vi "DO Control.vi"(9 "DI List_280":string[](array[string]), 10 "s":bool, 11 "DO":T1) -> (0 "Feedback":i32[](array[numeric]), 1 "Parameter (Out)":u8 caption="Poll Type", 2 "Control Channel 2":i32[](array[numeric]), 3 "Poll Time (Out)":u32 caption="Poll Time (ms)" max=600000 step=100, 4 "Value":enum32{"Output", "Input"}(ring), 5 "Cancel":bool)   [LabVIEW 2015]
uses:
  Control Button/Exit.ctl
  Control Button/next.ctl
  Control PB/output control.ctl
  Data Acquisition/PCI-USB-DAQ/Digital out put.ctl
  Galobal variable_TI.vi
panel:
  out "Row":i32
  in  "s 2":bool
  out "Pokayoka Result":cluster{"Sensor Name":string, "Boolean":bool}[](array[cluster]) caption="Pokayoka Status"
  in  "Tab Control":enum32{"Output", "Input"}(tab)
  in  "Control Channel":i32[](listbox)=[7]
  in  "op Add":T2
  in  "Feed Back Channel":i32[](listbox)=[0]
  in  "ok":T3
  in  "stop":T4
  # "Control Channel"
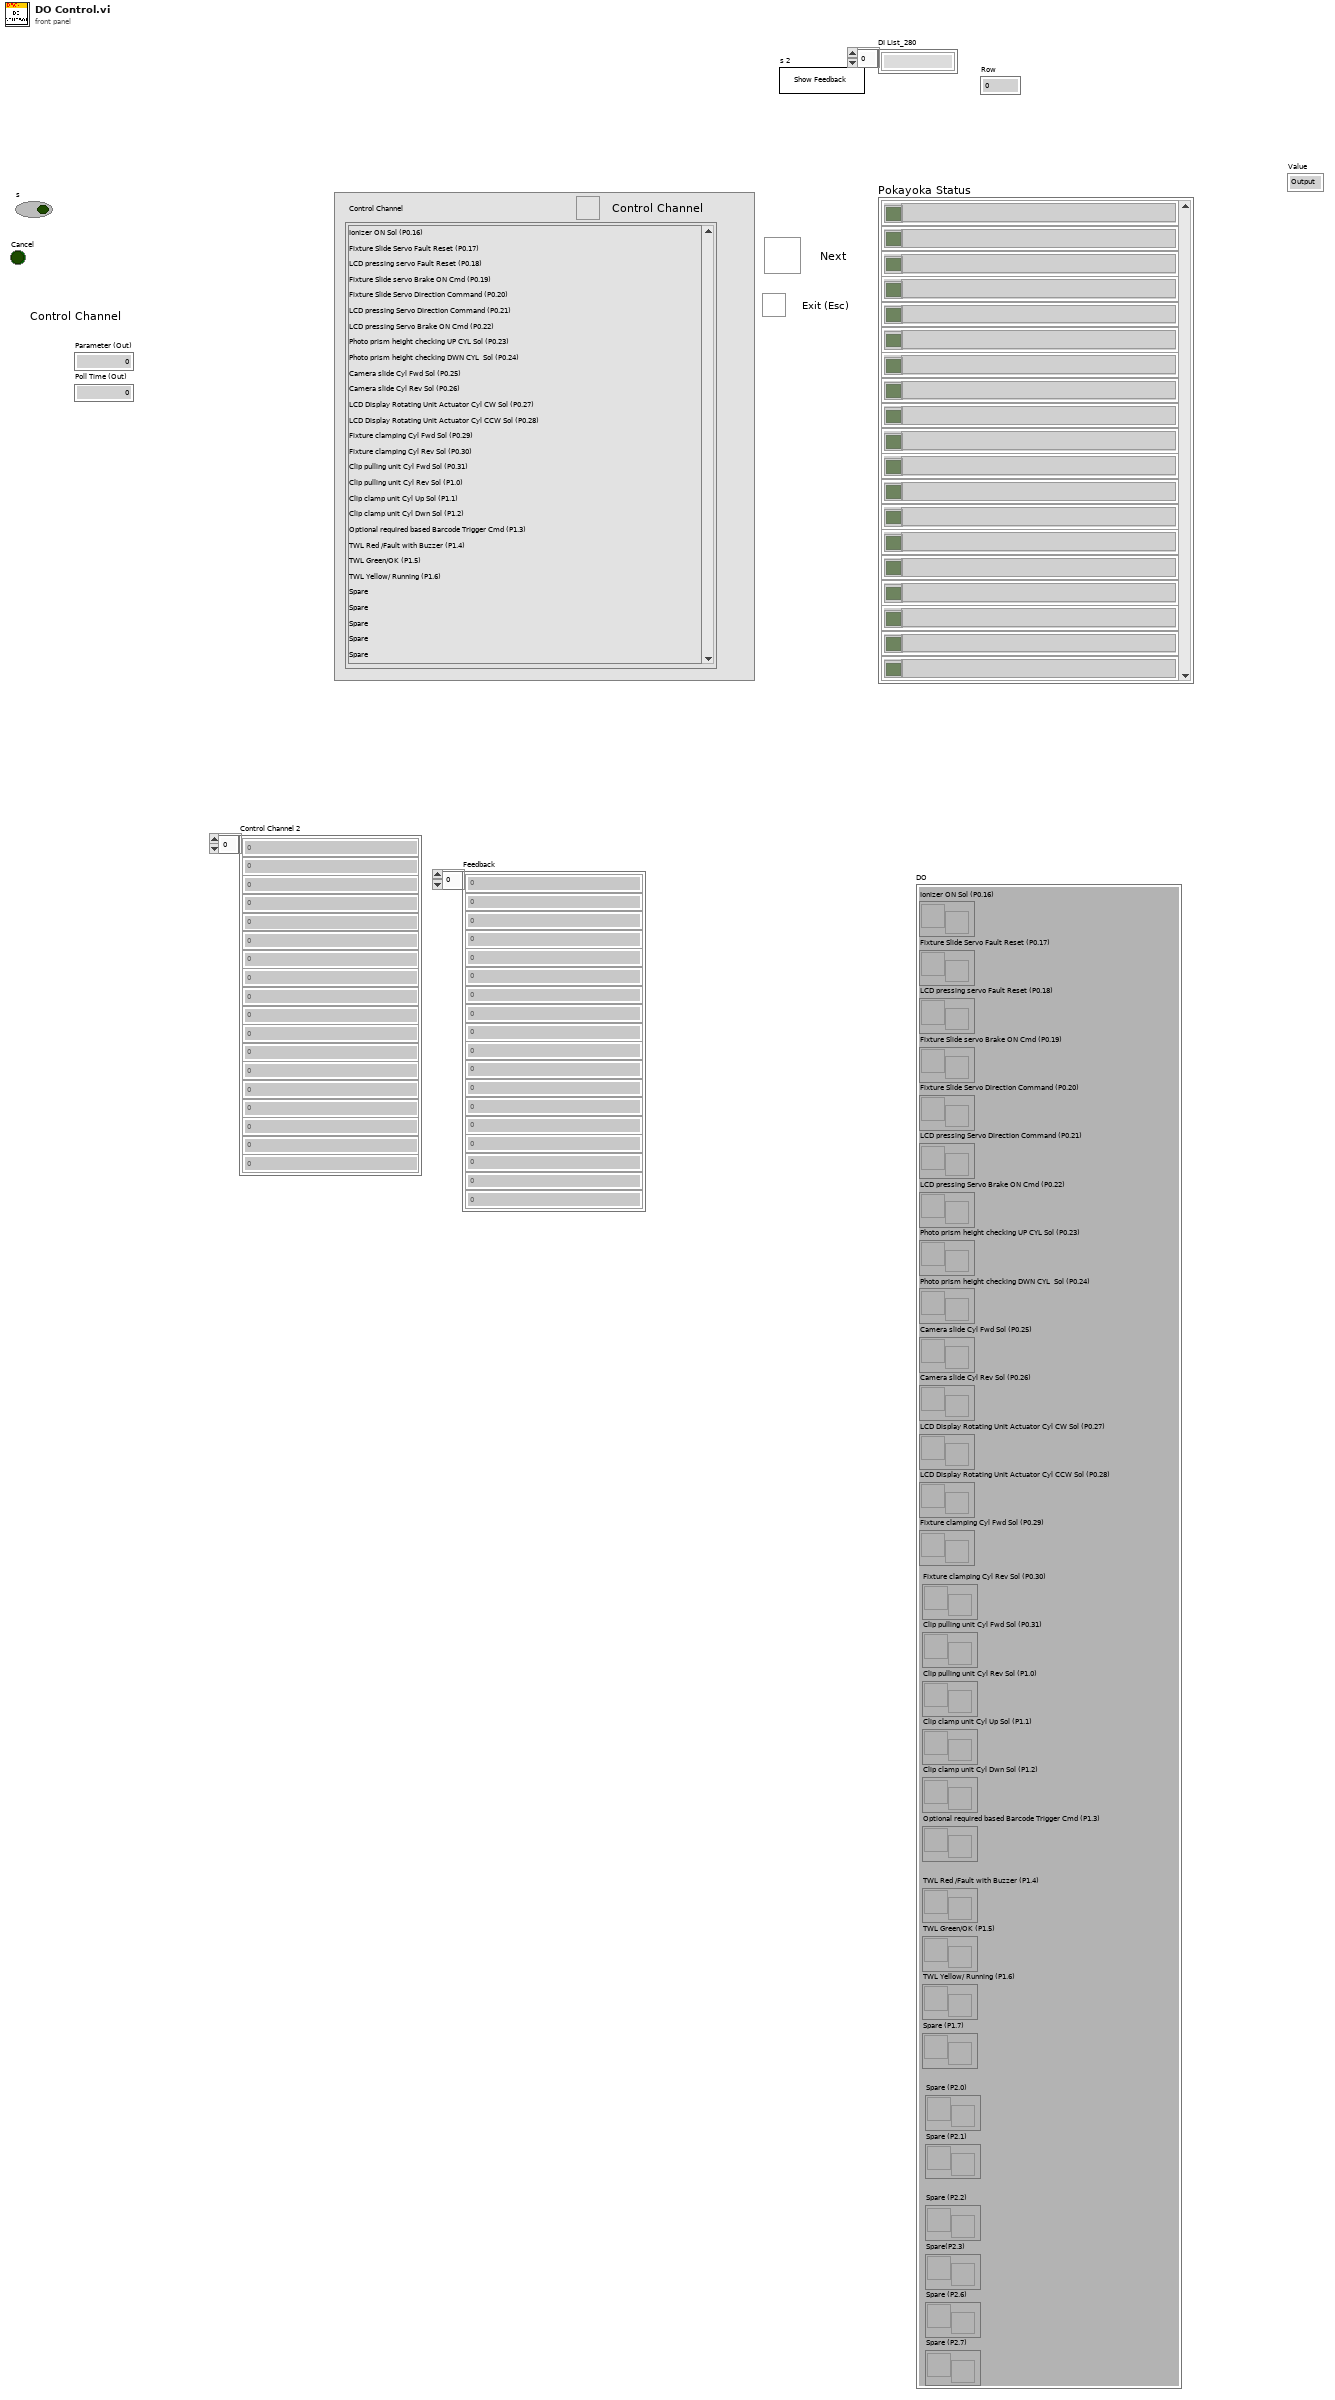
[diagram p1: front panel]
types:
  T1 = typedef "Digital out put.ctl" = cluster{"Ionizer ON Sol (P0.16)":refnum<notifier>, "Fixture Slide Servo Fault Reset (P0.17)":refnum<notifier>, "LCD pressing servo Fault Reset (P0.18)":refnum<notifier>, "Fixture Slide servo Brake ON Cmd (P0.19)":refnum<notifier>, "Fixture Slide Servo Direction Command (P0.20)":refnum<notifier>, "LCD pressing Servo Direction Command (P0.21)":refnum<notifier>, "LCD pressing Servo Brake ON Cmd (P0.22)":refnum<notifier>, "Photo prism height checking UP CYL Sol (P0.23)":refnum<notifier>, "Photo prism height checking DWN CYL  Sol (P0.24)":refnum<notifier>, "Camera slide Cyl Fwd Sol (P0.25)":refnum<notifier>, "Camera slide Cyl Rev Sol (P0.26)":refnum<notifier>, "LCD Display Rotating Unit Actuator Cyl CW Sol (P0.27)":refnum<notifier>, "LCD Display Rotating Unit Actuator Cyl CCW Sol (P0.28)":refnum<notifier>, "Fixture clamping Cyl Fwd Sol (P0.29)":refnum<notifier>, "Fixture clamping Cyl Rev Sol (P0.30)":refnum<notifier>, "Clip pulling unit Cyl Fwd Sol (P0.31)":refnum<notifier>, "Clip pulling unit Cyl Rev Sol (P1.0)":refnum<notifier>, "Clip clamp unit Cyl Up Sol (P1.1)":refnum<notifier>, "Clip clamp unit Cyl Dwn Sol (P1.2)":refnum<notifier>, "Optional required based Barcode Trigger Cmd (P1.3)":refnum<notifier>, "TWL Red /Fault with Buzzer (P1.4)":refnum<notifier>, "TWL Green/OK (P1.5)":refnum<notifier>, "TWL Yellow/ Running (P1.6)":refnum<notifier>, "Spare (P1.7)":refnum<notifier>, "Spare (P2.0)":refnum<notifier>, "Spare (P2.1)":refnum<notifier>, "Spare (P2.2)":refnum<notifier>, "Spare(P2.3)":refnum<notifier>, "Spare (P2.6)":refnum<notifier>, "Spare (P2.7) ":refnum<notifier>}
  T2 = typedef "output control.ctl" = bool
  T3 = typedef "next.ctl" = bool
  T4 = typedef "Exit.ctl" = bool
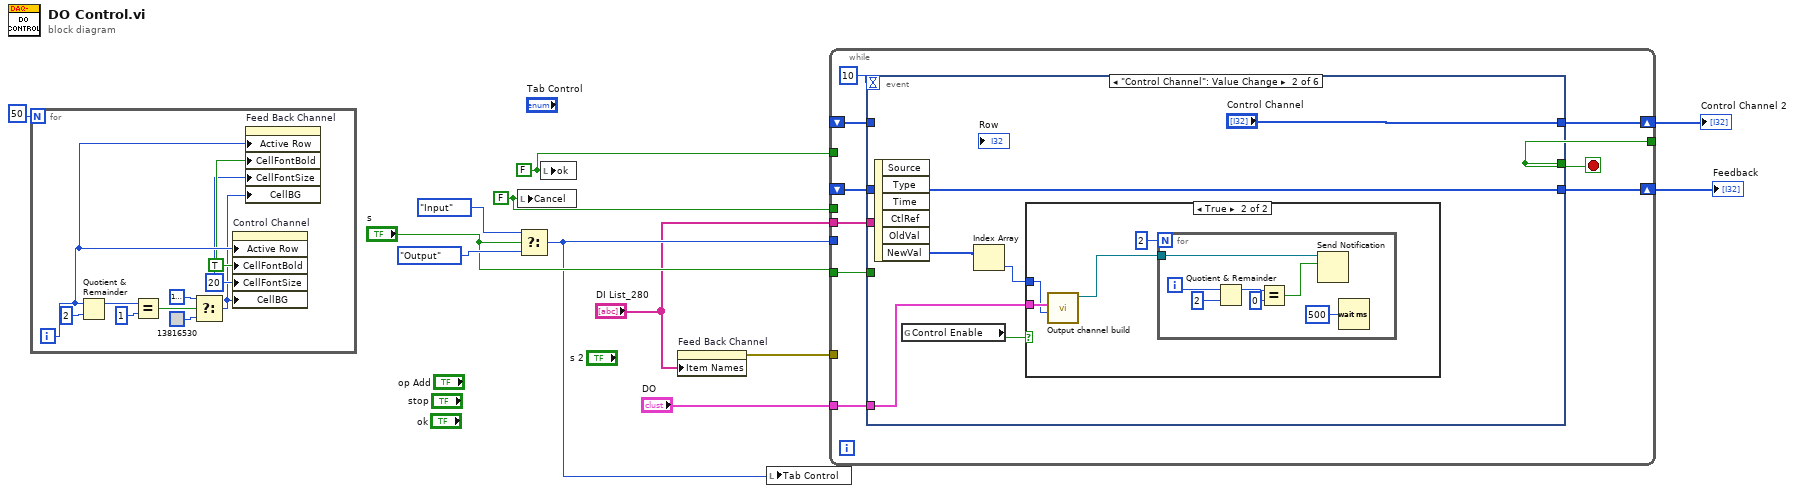
[diagram p0: block diagram]
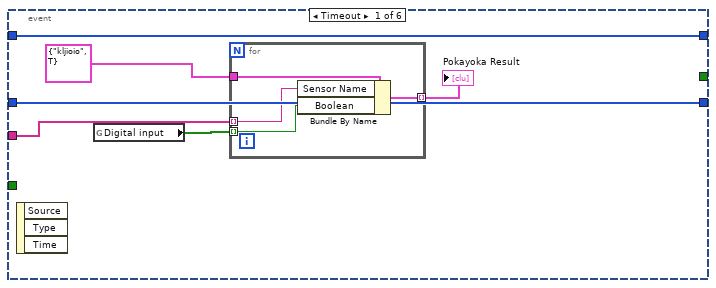
[diagram p2: hidden frame]
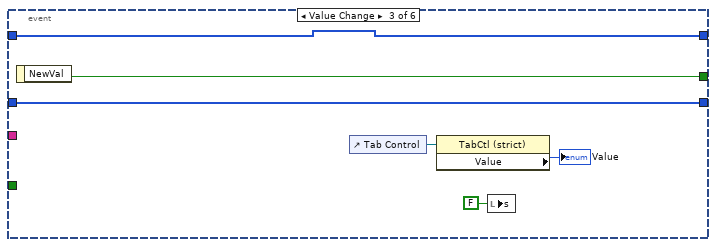
[diagram p4: hidden frame]
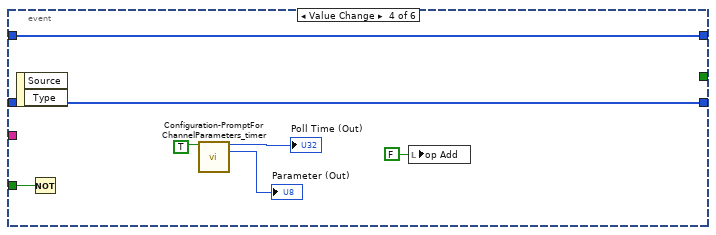
[diagram p5: hidden frame]
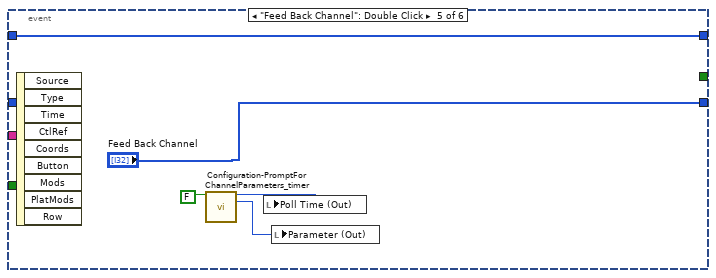
[diagram p6: hidden frame]
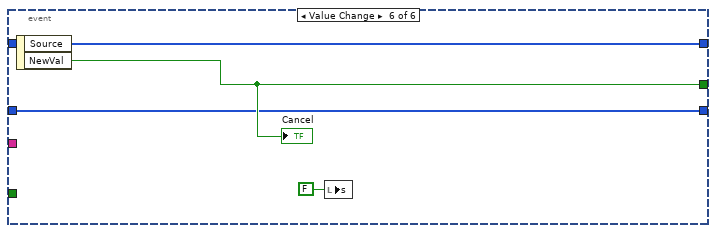
[diagram p7: hidden frame]
diagram:
  w5 = FALSE ("Cancel")
  w6 = FALSE ("ok")
  n1 = for {
    N: 50 -> [_]
    i -> [w16]
    w14 = u32 20 ("Active Row:Cell Font:Size")
    w15 = TRUE ("Active Row:Cell Font:Bold")
    n2 = Quotient & Remainder(x=w16, y=2) -> (x-y*floor(x/y)=w21:i32)  [unwired: 1 out]
    n3 = Equal?(x=w21, y=1) -> (x = y?=w19:bool)
    n4 = Select(t=u32 16777225 ("Color Box"), s=w19, f=u32 13816530 ("Color Box")) -> (s? t:f=w13:u32)
    n5 = property on="Control Channel" class="LstBox (strict)"("Active Row"=w16, "CellFontBold"=w15, "CellFontSize"=w14, "CellBG"=w13) -> ()  [unwired: 2 in, 2 out]
    n6 = property on="Feed Back Channel" class="LstBox (strict)"("Active Row"=w16, "CellFontBold"=w15, "CellFontSize"=w14, "CellBG"=w13) -> ()  [unwired: 2 in, 2 out]
  }
  n7 = local write "Cancel"(w5) -> ()
  n8 = Select(t=enum32{"Output", "Input"}."Input" ("Tab Control"), s="s", f=enum32{"Output", "Input"}."Output" ("Tab Control")) -> (s? t:f=w8:enum32{"Output", "Input"})
  n9 = local write "ok"(w6) -> ()
  n10 = property on="Feed Back Channel" class="LstBox (strict)"("Item Names"="DI List_280") -> (error out=w3:errorcluster)  [unwired: 2 in, 1 out]
  n11 = local write "Tab Control"(w8) -> ()
  n12 = while {
    tunnel: w8 -> [_]
    tunnel: "s" -> [w30]
    tunnel: w6 -> [_]
    tunnel: [w28] -> _
    tunnel: w5 -> [_]
    shift-right: [w31] -> w12
    shift-left: _ -> [w27]
    shift-right: [w29] -> w7
    shift-left: _ -> [w26]
    tunnel: "DI List_280" -> [w25]
    tunnel: w3 -> [_]
    tunnel: "DO" -> [w23]
    stop <- w28 stop-if-true
    n13 = event shown="[1] \"Control Channel\": Value Change" {
      selector: _ -> [_ _ _ _ _ _]
      dyn-events: _ -> [_ _ _ _ _ _]
      timeout: 10 -> [_ _ _ _ _ _]
      tunnel: [w37 "Control Channel" w60 w69 w73 w78] -> w31
      tunnel: [_ _ w64 _ _ w79] -> w28
      tunnel: w30 -> [_ _ _ w70 _ _]
      tunnel: [w36 w46 w59 w68 "Feed Back Channel" w77] -> w29
      tunnel: w27 -> [w37 _ w60 w69 w73 w78]
      tunnel: w26 -> [w36 w46 w59 w68 _ w77]
      tunnel: w25 -> [w33 _ _ _ _ _]
      tunnel: w23 -> [_ w43 _ _ _ _]
      event Timeout {
        n14 = event-data() -> ()  [unwired: 1 in, 3 out]
        n15 = global read "Galobal variable_TI.vi" "Digital input"() -> (w35:bool[])
        n16 = for {
          tunnel: w33 -> [w40] mode=indexing
          tunnel: cluster{"Sensor Name":string, "Boolean":bool} {"Sensor Name"="kljioio", "Boolean"=TRUE} ("Cluster") -> [w41]
          tunnel: [w39] -> w32 mode=indexing
          tunnel: w35 -> [w38] mode=indexing
          n17 = Bundle By Name(cluster=w41, "Sensor Name"=w40, "Boolean"=w38) -> (w39:cluster{"Sensor Name":string, "Boolean":bool})
        }
        "Pokayoka Result" <- w32
      }
      event "Control Channel": Value Change {
        n18 = event-data() -> ("NewVal"=w45:i32[])  [unwired: 1 in, 5 out]
        n19 = global read "Galobal variable_TI.vi" "Control Enable"() -> (w42:bool)
        n20 = Index Array(array=w45) -> (element=w44:i32)  [unwired: 1 in]
        n21 = case shown="True" w42 {
          tunnel: w44 -> [_ w50]
          tunnel: w43 -> [_ w51]
          frame False {
          }
          frame True {
            n22 = call "Output channel build.vi"("Channel No"=w50, "DO"=w51) -> ("Output channel"=w48:refnum<notifier>)  [unwired: 9 in]
            n23 = for {
              N: 2 -> [_]
              tunnel: w48 -> [w52]
              i -> [w58]
              n24 = Quotient & Remainder(x=w58, y=2) -> (x-y*floor(x/y)=w56:i32)  [unwired: 1 out]
              n25 = Equal?(x=w56, y=0) -> (x = y?=w54:bool)
              n26 = Send Notification(notification=w54, notifier=w52) -> ()  [unwired: 1 in, 2 out]
              n27 = Wait (ms)(milliseconds to wait=u32 500) -> ()  [unwired: 1 out]
            }
          }
        }
      }
      event Value Change {
        n28 = event-data() -> ("NewVal"=w64:T3)  [unwired: 1 in]
        n29 = control-ref of="Tab Control"() -> (w62:refnum<vi>)
        n30 = property class="TabCtl (strict)"(reference=w62) -> ("Value"=→"Value":enum32{"Output", "Input"})  [unwired: 1 in, 2 out]
        n31 = local write "s"(FALSE ("s")) -> ()
      }
      event Value Change {
        n32 = event-data() -> ()  [unwired: 1 in, 2 out]
        n33 = Not(x=w70) -> ()  [unwired: 1 out]
        n34 = call "Configuration-PromptForChannelParameters_timer.vi"("Control/Feedback\n(Default: False = Feedback)"=TRUE ("Control/Feedback\n(Default: False = Feedback)")) -> ("Poll Time (Out)"=→"Poll Time (Out)":u32, "Parameter (Out)"=→"Parameter (Out)":u8)  [unwired: 13 in]
        n35 = local write "op Add"(T2 FALSE ("op Add")) -> ()
      }
      event "Feed Back Channel": Double Click {
        n36 = event-data() -> ()  [unwired: 1 in, 9 out]
        n37 = call "Configuration-PromptForChannelParameters_timer.vi"("Control/Feedback\n(Default: False = Feedback)"=FALSE ("Control/Feedback\n(Default: False = Feedback)")) -> ("Poll Time (Out)"=w75:u32, "Parameter (Out)"=w74:u8)  [unwired: 13 in]
        n38 = local write "Poll Time (Out)"(w75) -> ()
        n39 = local write "Parameter (Out)"(w74) -> ()
      }
      event Value Change {
        n40 = event-data() -> ("NewVal"=w79:T4)  [unwired: 1 in, 1 out]
        "Cancel" <- w79
        n41 = local write "s"(FALSE ("s")) -> ()
      }
    }
  }
  "Control Channel 2" <- w12
  "Feedback" <- w7
